vi "Test_Aquisition_Reactor_Coolant_Loop_Temperature_SG_Outlet.vi"() -> ()   [LabVIEW 2022 SP3]
uses:
  SI_modules/SI101/SI101.lvclass
panel:
  out "Avg Temp rise":cluster{"Time":timestamp[], dbl[]}[](graph)
  out "Inputs":cluster{"Time":timestamp[], dbl[]}[](graph)
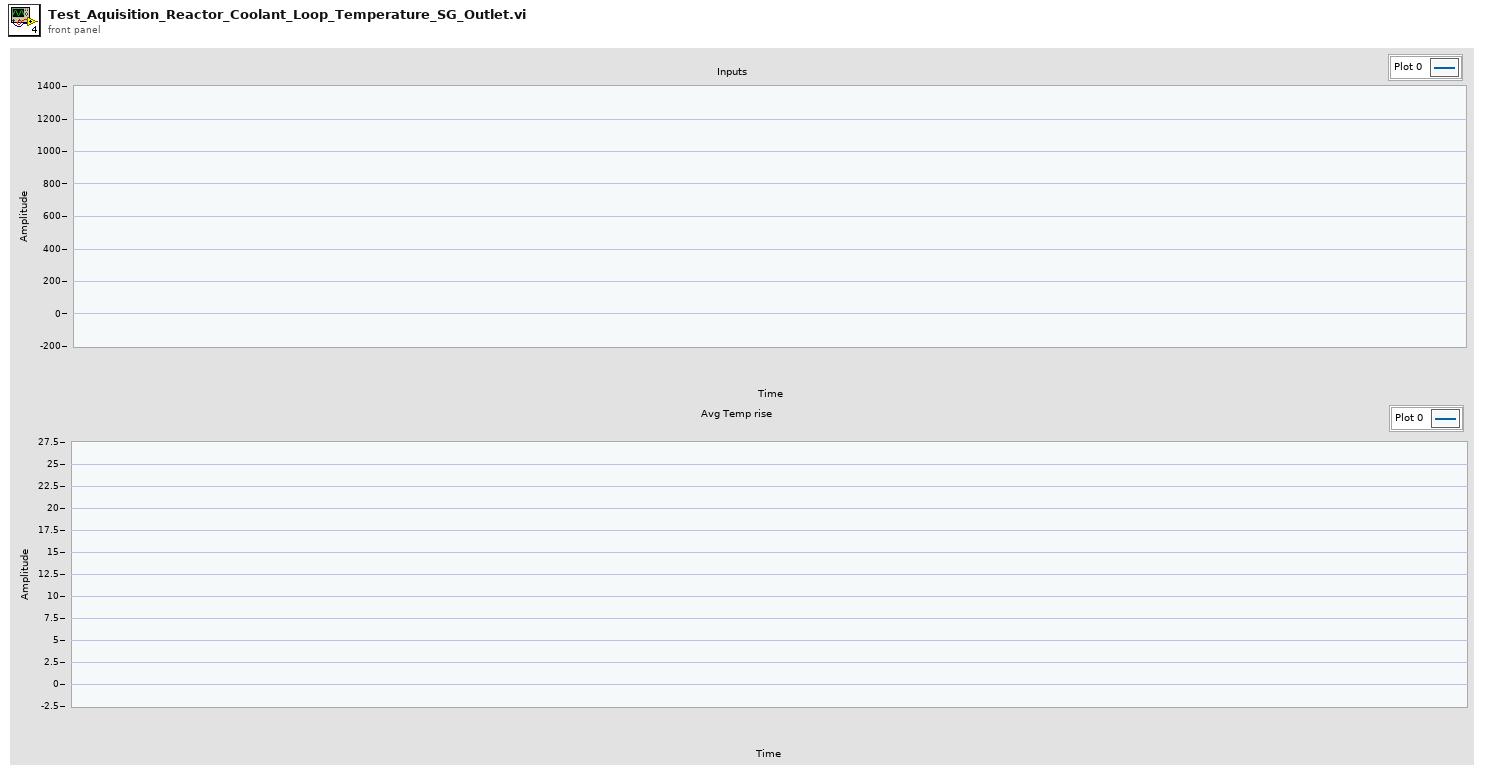
[diagram p1: front panel]
types:
  T1 = cluster{"[0]":cluster{"Time":timestamp[], "KKS":string, "Meas":dbl[]}, "[1]":cluster{"Time":timestamp[], "KKS":string, "Meas":dbl[]}, "[2]":cluster{"Time":timestamp[], "KKS":string, "Meas":dbl[]}, "[3]":cluster{"Time":timestamp[], "KKS":string, "Meas":dbl[]}, "[4]":cluster{"Time":timestamp[], "KKS":string, "Meas":dbl[]}, "[5]":cluster{"Time":timestamp[], "KKS":string, "Meas":dbl[]}, "[6]":cluster{"Time":timestamp[], "KKS":string, "Meas":dbl[]}, "[7]":cluster{"Time":timestamp[], "KKS":string, "Meas":dbl[]}, "[8]":cluster{"Time":timestamp[], "KKS":string, "Meas":dbl[]}}
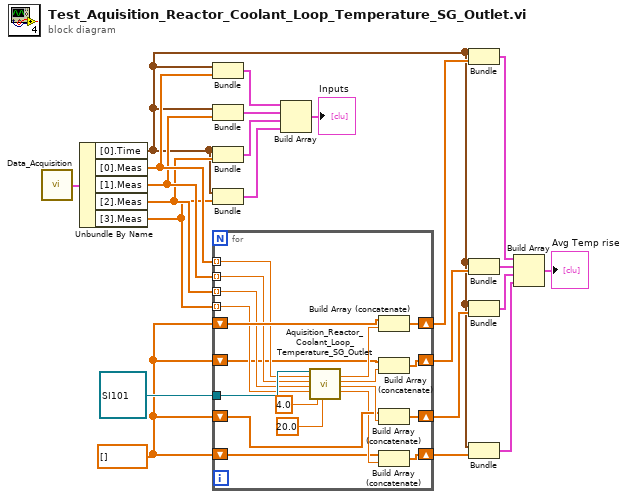
[diagram p0: block diagram]
diagram:
  w10 = dbl[] []
  n1 = call "Data_Acquisition.vi"() -> ("Meas"=w22:T1)  [unwired: 15 in]
  n2 = Unbundle By Name(w22) -> ("[0].Time"=w7:timestamp[], "[0].Meas"=w21:dbl[], "[1].Meas"=w20:dbl[], "[2].Meas"=w19:dbl[], "[3].Meas"=w18:dbl[])
  n3 = Bundle("Time"=w7, "Meas"=w21) -> (w17:cluster{"Time":timestamp[], "Meas":dbl[]})  [unwired: 1 in]
  n4 = Bundle("Time"=w7, "Meas"=w20) -> (w16:cluster{"Time":timestamp[], "Meas":dbl[]})  [unwired: 1 in]
  n5 = Bundle("Time"=w7, "Meas"=w19) -> (w15:cluster{"Time":timestamp[], "Meas":dbl[]})  [unwired: 1 in]
  n6 = Bundle("Time"=w7, "Meas"=w18) -> (w14:cluster{"Time":timestamp[], "Meas":dbl[]})  [unwired: 1 in]
  n7 = for {
    tunnel: w21 -> [w39] mode=indexing
    tunnel: w20 -> [w38] mode=indexing
    tunnel: w19 -> [w37] mode=indexing
    tunnel: w18 -> [w36] mode=indexing
    shift-right: [w29] -> w12
    shift-left: w10 -> [w41]
    tunnel: refnum<class "SI101.lvclass"> refnum ("SI101_AverageReactorCoolantTemperature.lvclass") -> [w40]
    shift-right: [w30] -> w9
    shift-left: w10 -> [w31]
    shift-right: [w27] -> w8
    shift-left: w10 -> [w26]
    shift-right: [w24] -> w6
    shift-left: w10 -> [w23]
    n8 = call "Aquisition_Reactor_Coolant_Loop_Temperature_SG_Outlet.vi"("SI101_AverageReactorCoolantTemperature.lvclass"=w40, "3 JEC10 CT001A XQ01"=w39, "3 JEC20 CT001A XQ01"=w38, "3 JEC30 CT001A XQ01"=w37, "3 JEC40 CT001A XQ01"=w36, "In1"=4.0, "In2"=20.0) -> ("JEC10CT001A"=w33:dbl, "JEC20CT001A"=w32:dbl, "JEC30CT001A"=w28:dbl, "JEC40CT001A"=w25:dbl)  [unwired: 7 in, 2 out]
    n9 = Build Array (concatenate)(w41, w33) -> (w29:dbl[])
    n10 = Build Array (concatenate)(w31, w32) -> (w30:dbl[])
    n11 = Build Array (concatenate)(w26, w28) -> (w27:dbl[])
    n12 = Build Array (concatenate)(w23, w25) -> (w24:dbl[])
  }
  n13 = Build Array(w17, w16, w15, w14) -> (→"Inputs":cluster{"Time":timestamp[], "Meas":dbl[]}[])
  n14 = Bundle("Time"=w7, w12) -> (w5:cluster{"Time":timestamp[], dbl[]})  [unwired: 1 in]
  n15 = Bundle("Time"=w7, w9) -> (w4:cluster{"Time":timestamp[], dbl[]})  [unwired: 1 in]
  n16 = Bundle("Time"=w7, w8) -> (w3:cluster{"Time":timestamp[], dbl[]})  [unwired: 1 in]
  n17 = Bundle("Time"=w7, w6) -> (w2:cluster{"Time":timestamp[], dbl[]})  [unwired: 1 in]
  n18 = Build Array(w5, w4, w3, w2) -> (→"Avg Temp rise":cluster{"Time":timestamp[], dbl[]}[])
